vi "Handle.vi"(7 "Queue jettl in":refnum<class "Queue Actor.lvclass">, 11 "Teardown State in":refnum<class "Teardown State.lvclass">) -> (2 "Destroy?":bool, 5 "Queue jettl out":refnum<class "Queue Actor.lvclass">)   [LabVIEW 2021, in "jettl.lvlib" / "Base Queue jettl.lvlib" / "Teardown State.lvclass"]
uses:
  Teardown State.lvclass
  Queue Actor/Queue Actor.lvclass
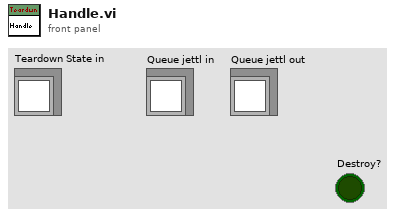
[diagram p1: front panel]
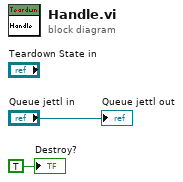
[diagram p0: block diagram]
diagram:
  "Destroy?" <- TRUE ("Destroy?")
  "Queue jettl out" <- "Queue jettl in"
